vi "Circle1005.vi"   [LabVIEW 2013]
uses:
  <vilib>/Heliosphere Research LLC/Advanced Plotting Toolkit/api_core/NewPlotProperties.ctl
  <vilib>/Heliosphere Research LLC/Advanced Plotting Toolkit/typedefs/PlotColor.ctl
  <vilib>/Heliosphere Research LLC/Advanced Plotting Toolkit/api_annotations/ShapeProperties.ctl
  <vilib>/Heliosphere Research LLC/Advanced Plotting Toolkit/properties/Line.ctl
  <vilib>/Heliosphere Research LLC/Advanced Plotting Toolkit/properties/Line_Style.ctl
  <vilib>/Heliosphere Research LLC/Advanced Plotting Toolkit/properties/Display.ctl
  <vilib>/Heliosphere Research LLC/Advanced Plotting Toolkit/Advanced Plotting Toolkit.lvlib
types:
  T1 = typedef "Advanced Plotting Toolkit.lvlib/ShapeProperties.ctl" = cluster{"Color":T2, "Line":T3, "Display":T5}
  T2 = typedef "Advanced Plotting Toolkit.lvlib/PlotColor.ctl" = u32
  T3 = typedef "Advanced Plotting Toolkit.lvlib/Line.ctl" = cluster{"Style":T4, "Color":T2, "Width":sgl}
  T4 = typedef "Advanced Plotting Toolkit.lvlib/Line_Style.ctl" = enum16{"Automatic", "Solid", "Dashed", "Dotted", "Dash-dot", "Invisible"}
  T5 = typedef "Advanced Plotting Toolkit.lvlib/Display.ctl" = cluster{"Alpha":dbl, "Z Order":dbl}
  T6 = typedef "Advanced Plotting Toolkit.lvlib/NewPlotProperties.ctl" = cluster{"Background Color":T2, "Axis Background":T2, "Left Margin":dbl, "Right Margin":dbl, "Bottom Margin":dbl, "Top Margin":dbl, "Aspect Ratio":dbl}
  T7 = typedef "Advanced Plotting Toolkit.lvlib/PlotID.ctl" = i32
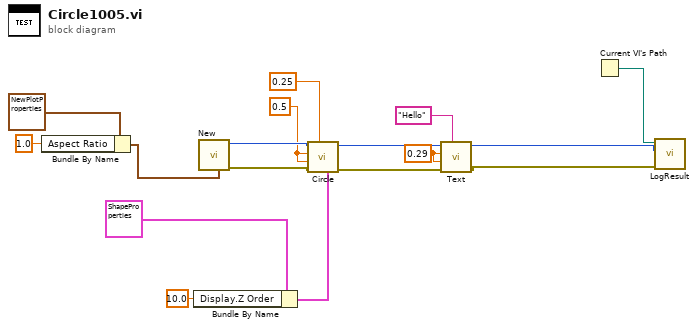
[diagram p0: block diagram]
diagram:
  w1 = 0.29 ("X Position")
  w3 = 0.5 ("X Position")
  n1 = Bundle By Name(cluster=T6 {"Background Color"=2147483647, "Axis Background"=2147483647, "Left Margin"=nan, "Right Margin"=nan, "Bottom Margin"=nan, "Top Margin"=nan, "Aspect Ratio"=nan} ("New Plot Properties"), "Aspect Ratio"=1.0) -> (w13:T6)
  n2 = Bundle By Name(cluster=T1 {"Color"=2147483647, "Line"={"Style"=enum."Automatic", "Color"=2147483647, "Width"=nan}, "Display"={"Alpha"=nan, "Z Order"=nan}} ("Shape Properties"), "Display.Z Order"=10.0 ("Display.Alpha")) -> (w9:T1)
  n3 = call <vilib>:"New.vi"("Properties"=w13) -> ("error out"=w15:errorcluster, "Plot ID"=w16:T7)  [unwired: 9 in]
  n4 = call <vilib>:"Circle.vi"("Properties"=w9, "Radius"=0.25, "error in (no error)"=w15, "Y Position"=w3, "X Position"=w3, "Plot ID"=w16) -> ("error out"=w4:errorcluster, "Plot ID Out"=w7:T7)  [unwired: 4 in]
  n5 = call <vilib>:"Text.vi"("Text"="Hello", "error in (no error)"=w4, "Y Position"=w1, "X Position"=w1, "Plot ID"=w7) -> ("error out"=w5:errorcluster, "Plot ID Out"=w6:T7)  [unwired: 5 in]
  n6 = Current VI's Path() -> (path=w17:path)
  n7 = call "LogResult.vi"("Test Result"=w5, "Test Artifact"=w6, "VI Path"=w17) -> ()  [unwired: 9 in]
